vi "PQ Test Invalid User.vi"(8 "error in (no error)":errorcluster, 10 "Connection String":string="user = llab_read") -> (0 "error out":errorcluster)   [LabVIEW 2019]
uses:
  <vilib>/addons/_JKI Toolkits/Caraya/classes/Assert/Assert Error.vi
  src/LV-Data.PG/LV-Data.PGSQL.lvclass
  <vilib>/addons/_JKI Toolkits/Caraya/classes/Assert/Assert.lvclass
  <vilib>/addons/_JKI Toolkits/Caraya/classes/Test/Test.lvclass
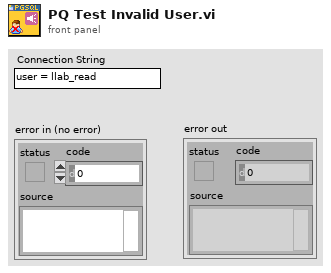
[diagram p1: front panel]
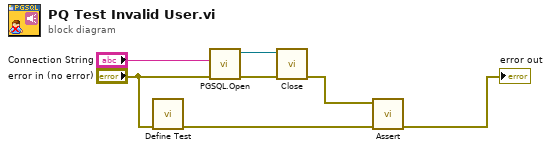
[diagram p0: block diagram]
diagram:
  n1 = call <vilib>:"Define Test.vi"("error in (no error)"="error in (no error)") -> ("error out"=w1:errorcluster)  [unwired: 9 in, 1 out]
  n2 = call "PGSQL.Open.vi"("error in (no error)"="error in (no error)", "Connection String"="Connection String") -> ("error out"=w7:errorcluster, "Data.PG out"=w6:refnum<class "LV-Data.PGSQL.lvclass">)  [unwired: 8 in]
  n3 = call-dynamic "Close.vi"("error in (no error)"=w7, "Data.PG in"=w6) -> ("error out"=w4:errorcluster)  [unwired: 8 in, 1 out]
  n4 = call-poly <vilib>:"Assert.vi"("error in (no error)"=w1, "Error?"=w4) -> ("error out"=→"error out":errorcluster)  [unwired: 8 in, 1 out]
